vi "Set Expected Channel Count.vi"(8 "error in":errorcluster, 11 "module test in":refnum<class "Module Test.lvclass">) -> (0 "error out":errorcluster, 3 "module test out":refnum<class "Module Test.lvclass">)   [LabVIEW 2017, in "Module Test.lvclass"]
uses:
  Module Test.lvclass
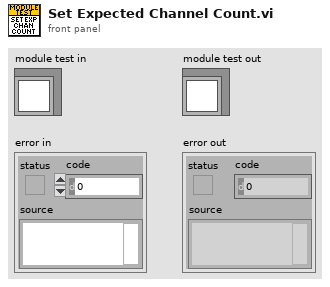
[diagram p1: front panel]
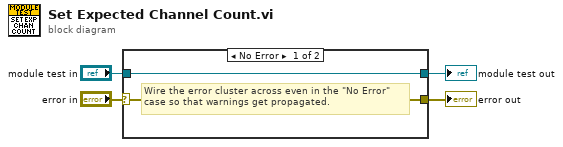
[diagram p0: block diagram]
diagram:
  n1 = case shown="No Error" "error in" {
    selector: "error in" -> [w5 w8]
    tunnel: [w5 w8] -> w3
    tunnel: [w6 w7] -> w1
    tunnel: "module test in" -> [w6 w7]
    frame No Error {
      # "Wire the error cluster across even in the \"No Error\"\ncase so that warnings get propagated."
    }
    frame Error {
    }
  }
  "error out" <- w3
  "module test out" <- w1
